vi "Data stream reader global.vi"() -> ()   [LabVIEW 2015]
panel:
  out "Data stream reader":refnum<k21>
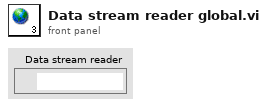
[diagram p1: front panel]
diagram:
